vi "Dig Grave Target.vi"(11 "Boolean":bool=TRUE) -> (3 "Cluster":cluster{string, i32})   [LabVIEW 2017, in "Tests.lvlib"]
uses:
  Tests.lvlib
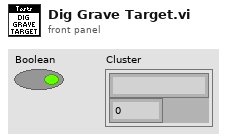
[diagram p1: front panel]
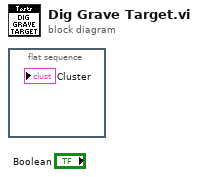
[diagram p0: block diagram]
diagram:
  n1 = flat-sequence {
    frame #0 {
    }
  }
